vi "Divideby3.vi"(1 "C":i16, 2 "B":i16, 3 "A":i16) -> (0 "Divideby3":i16)   [LabVIEW 2016]
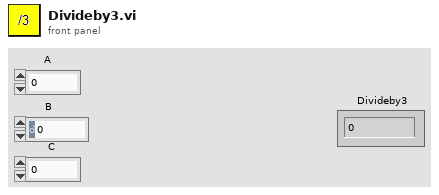
[diagram p1: front panel]
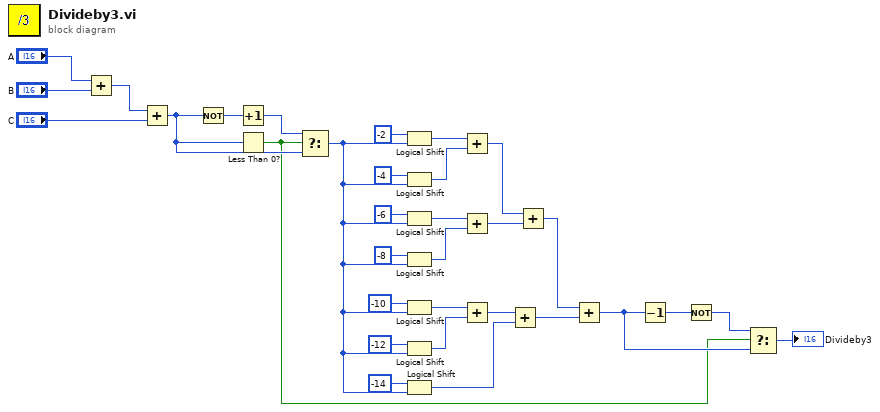
[diagram p0: block diagram]
diagram:
  n1 = Add(x="A", y="B") -> (x+y=w31:i16)
  n2 = Add(x=w31, y="C") -> (x+y=w9:i16)
  n3 = Not(x=w9) -> (.not. x?=w8:i16)
  n4 = Increment(x=w8) -> (x+1=w7:i16)
  n5 = Less Than 0?(x=w9) -> (x < 0?=w3:bool)
  n6 = Select(t=w7, s=w3, f=w9) -> (s? t:f=w6:i16)
  n7 = Logical Shift(y=i16 -2, x=w6) -> (x << y=w16:i16)
  n8 = Logical Shift(y=i16 -4, x=w6) -> (x << y=w15:i16)
  n9 = Logical Shift(y=i16 -6, x=w6) -> (x << y=w14:i16)
  n10 = Logical Shift(y=i16 -8, x=w6) -> (x << y=w13:i16)
  n11 = Logical Shift(y=i16 -10, x=w6) -> (x << y=w12:i16)
  n12 = Logical Shift(y=i16 -12, x=w6) -> (x << y=w11:i16)
  n13 = Logical Shift(y=i16 -14, x=w6) -> (x << y=w10:i16)
  n14 = Add(x=w16, y=w15) -> (x+y=w22:i16)
  n15 = Add(x=w14, y=w13) -> (x+y=w21:i16)
  n16 = Add(x=w12, y=w11) -> (x+y=w20:i16)
  n17 = Add(x=w20, y=w10) -> (x+y=w18:i16)
  n18 = Add(x=w22, y=w21) -> (x+y=w19:i16)
  n19 = Add(x=w19, y=w18) -> (x+y=w4:i16)
  n20 = Decrement(x=w4) -> (x-1=w1:i16)
  n21 = Not(x=w1) -> (.not. x?=w2:i16)
  n22 = Select(t=w2, s=w3, f=w4) -> (s? t:f=→"Divideby3":i16)
